vi "Lian_Lab07_II.vi"() -> ()   [LabVIEW 2020]
uses:
  <vilib>/DAQmx/read.llb/DAQmx Read (Counter DBL 1Chan 1Samp).vi
  <vilib>/DAQmx/create/channels.llb/DAQmx Create Channel (CI-Count Edges).vi
  <vilib>/DAQmx/miscellaneous.llb/DAQmx Fill In Error Info.vi
panel:
  out "Waveform Chart":dbl(graph)
  in  "?":bool
  in  "Loop Delay (ms)":u32
  in  "Counter Channel":tag
  # "Part II."
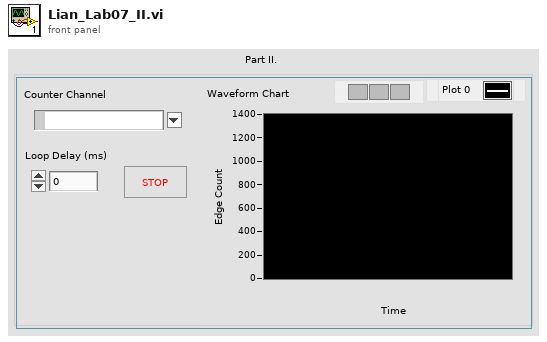
[diagram p1: front panel]
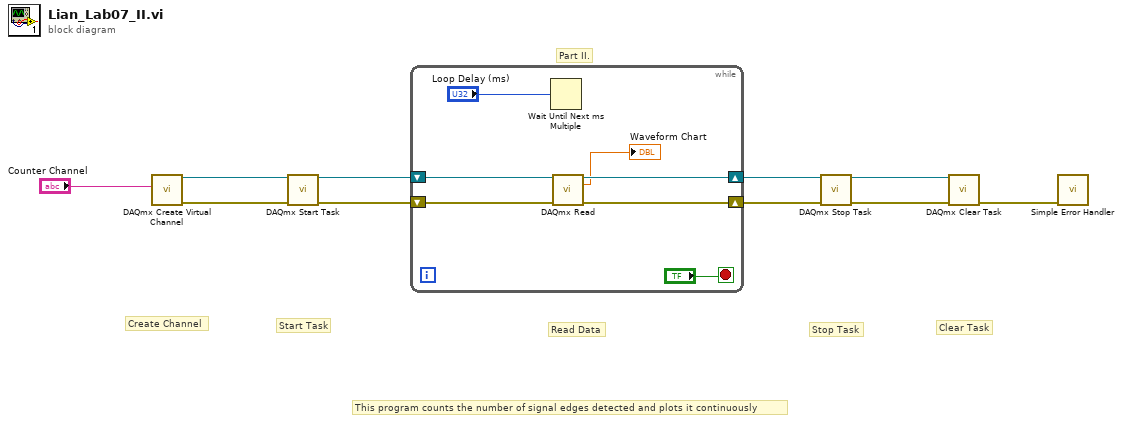
[diagram p0: block diagram]
diagram:
  # "This program counts the number of signal edges detected and plots it continuously"
  # "Read Data"
  # "Clear Task"
  # "Stop Task"
  # "Start Task"
  # "Create Channel"
  # "Part II."
  n1 = call-poly <vilib>:"DAQmx Create Virtual Channel.vi"("counter"="Counter Channel") -> ("task out"=w2:refnum<k21>, "error out"=w1:errorcluster)  [unwired: 13 in]
  n2 = call <vilib>:"DAQmx Start Task.vi"("task/channels in"=w2, "error in"=w1) -> ("task out"=w4:refnum<k21>, "error out"=w3:errorcluster)  [unwired: 12 in]
  n3 = while {
    shift-right: [w17] -> w10
    shift-left: w4 -> [w15]
    shift-right: [w16] -> w6
    shift-left: w3 -> [w14]
    stop <- "?" stop-if-true
    n4 = Wait Until Next ms Multiple(millisecond multiple="Loop Delay (ms)") -> ()  [unwired: 1 out]
    n5 = call-poly <vilib>:"DAQmx Read.vi"("task/channels in"=w15, "error in"=w14) -> ("task out"=w17:refnum<k21>, "data"=→"Waveform Chart":dbl, "error out"=w16:errorcluster)  [unwired: 11 in]
  }
  n6 = call <vilib>:"DAQmx Stop Task.vi"("task/channels in"=w10, "error in"=w6) -> ("task out"=w9:refnum<k21>, "error out"=w7:errorcluster)  [unwired: 12 in]
  n7 = call <vilib>:"DAQmx Clear Task.vi"("task in"=w9, "error in"=w7) -> ("error out"=w8:errorcluster)  [unwired: 13 in]
  n8 = call <vilib>:"Simple Error Handler.vi"("error in (no error)"=w8) -> ()  [unwired: 4 in, 5 out]
